vi "Config.vi"() -> ()   [LabVIEW 2020]
uses:
  Global_Variable/Global.vi
  <vilib>/Utility/config.llb/NI_LVConfig.lvlib
  Libraries/S7/S7.lvlib
panel:
  in  "扭矩偏移":string[][](table)=[["mm"], ["mm/s"], ["mm"], ["mm/s"]]
  in  "选项卡控件":enum32{"输入轴", "静态标定", "可信度检测", "传感器特性"}(tab)
  in  "左工位输入轴参数":string[][](table)=[["mm"], ["mm/s"], ["mm"], ["mm/s"]]
  in  "右工位输入轴参数":string[][](table)=[["mm"], ["mm/s"], ["mm"], ["mm/s"]]
  in  "静态标定判定":string[][](table)=[["mm"], ["mm/s"], ["mm"], ["mm/s"]]
  in  "跳过优化":bool
  in  "8点复测":bool
  in  "动态优化复测":bool
  in  "可信度检测参数":string[][](table)=[["mm/s"], ["°"], ["mm/s"]]
  in  "动态优化判定":string[][](table)=[["%"], ["%"], ["%"], ["%"]]
  in  "复检参数":string[][](table)=[["°/s"], ["Nm"], ["°"], ["°"], ["°"], ["°"]]
  in  "判定参数":string[][](table)=[["%", "", ""], ["%", "", ""], ["%", "", ""], ["%", "", ""], ["%", "", ""], ["%", "", ""], ["%", "", ""], ["%", "", ""], ["%", "", ""], ["Nm", "", ""], ["%", "", ""], ["%", "", ""], ["%", "", ""], ["%", "", ""]]
  in  "可信度检测":bool
  in  "传感器特性":bool
  in  "程序固化":bool
  in  "静态标定":bool
  in  "产品型号":string(combo)
  in  "删除":bool
  in  "确定":bool
  in  "添加":bool
  in  "退出":bool
  in  "更新":bool
  # "传感器对中台"
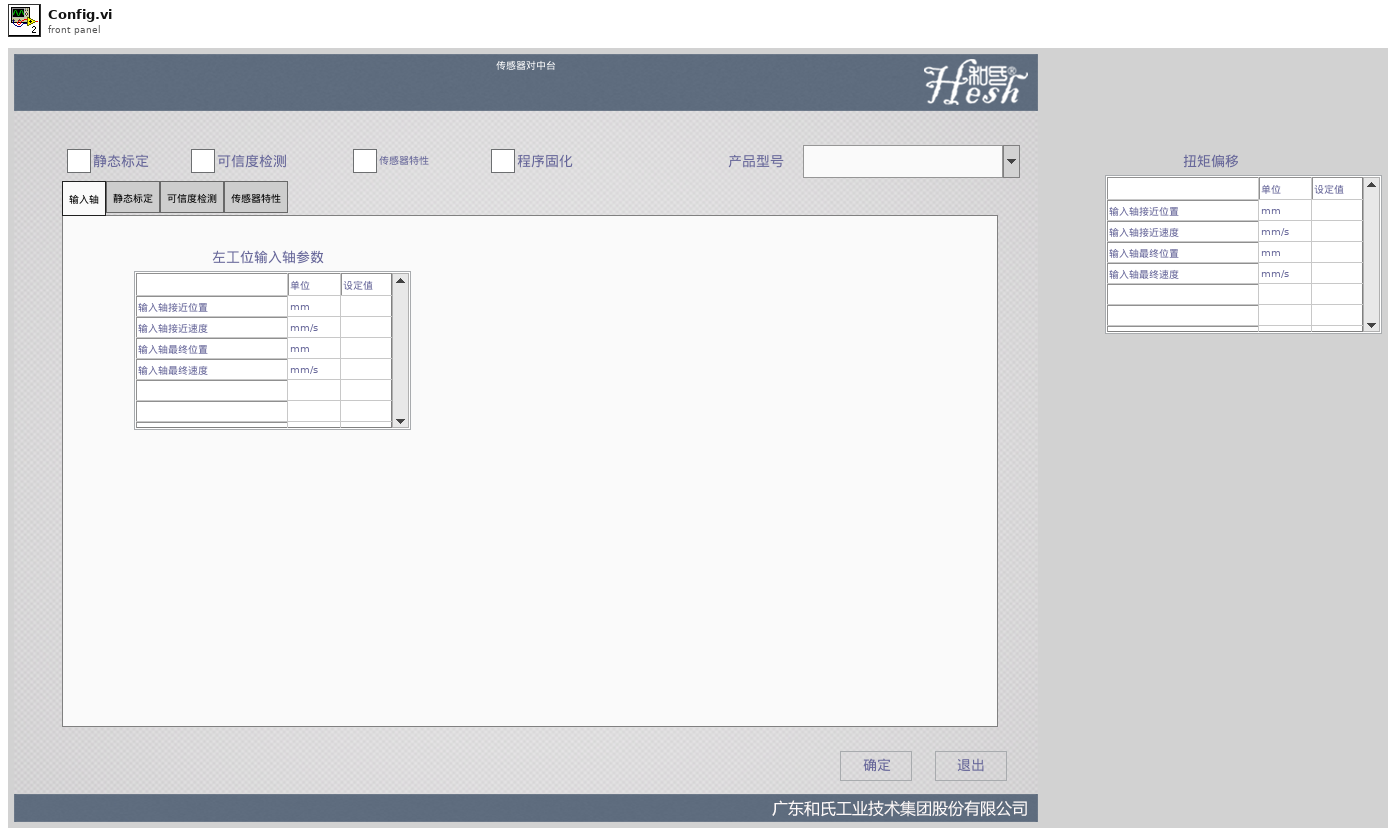
[diagram p1: front panel]
types:
  T1 = enum8{"Enabled", "Disabled", "Disabled and Grayed Out"}
  T2 = typedef "检测CTR.xctl/检测CTR数据.ctl" = enum16{"Idle", "Runing", "Pass", "Faild", "Skip"}
  T3 = cluster{"操作员编号":string, "操作员姓名":string, "操作员权限":string, "联机模式":enum16{"单机", "追溯"}}
  T4 = typedef "NI_LVConfig.lvlib/Config Data RefNum.ctl" = refnum<k1>
  T5 = cluster{"[0]":cluster{string, dbl, dbl}, "[1]":cluster{string, dbl, dbl}, "[2]":cluster{string, dbl, dbl}, "[3]":cluster{string, dbl, dbl}, "[4]":cluster{string, dbl, dbl}}
  T6 = cluster{"[0]":dbl, "[1]":dbl, "[2]":dbl, "[3]":dbl, "[4]":dbl, "[5]":dbl, "[6]":dbl}
  T7 = cluster{"[0]":cluster{string, dbl, dbl}, "[1]":cluster{string, dbl, dbl}, "[2]":cluster{string, dbl, dbl}, "[3]":cluster{string, dbl, dbl}, "[4]":cluster{string, dbl, dbl}, "[5]":cluster{string, dbl, dbl}, "[6]":cluster{string, dbl, dbl}, "[7]":cluster{string, dbl, dbl}, "[8]":cluster{string, dbl, dbl}, "[9]":cluster{string, dbl, dbl}, "[10]":cluster{string, dbl, dbl}, "[11]":cluster{string, dbl, dbl}, "[12]":cluster{string, dbl, dbl}, "[13]":cluster{string, dbl, dbl}, "[14]":cluster{string, dbl, dbl}, "[15]":cluster{string, dbl, dbl}, "[16]":cluster{string, dbl, dbl}, "[17]":cluster{string, dbl, dbl}, "[18]":cluster{string, dbl, dbl}, "[19]":cluster{string, dbl, dbl}}
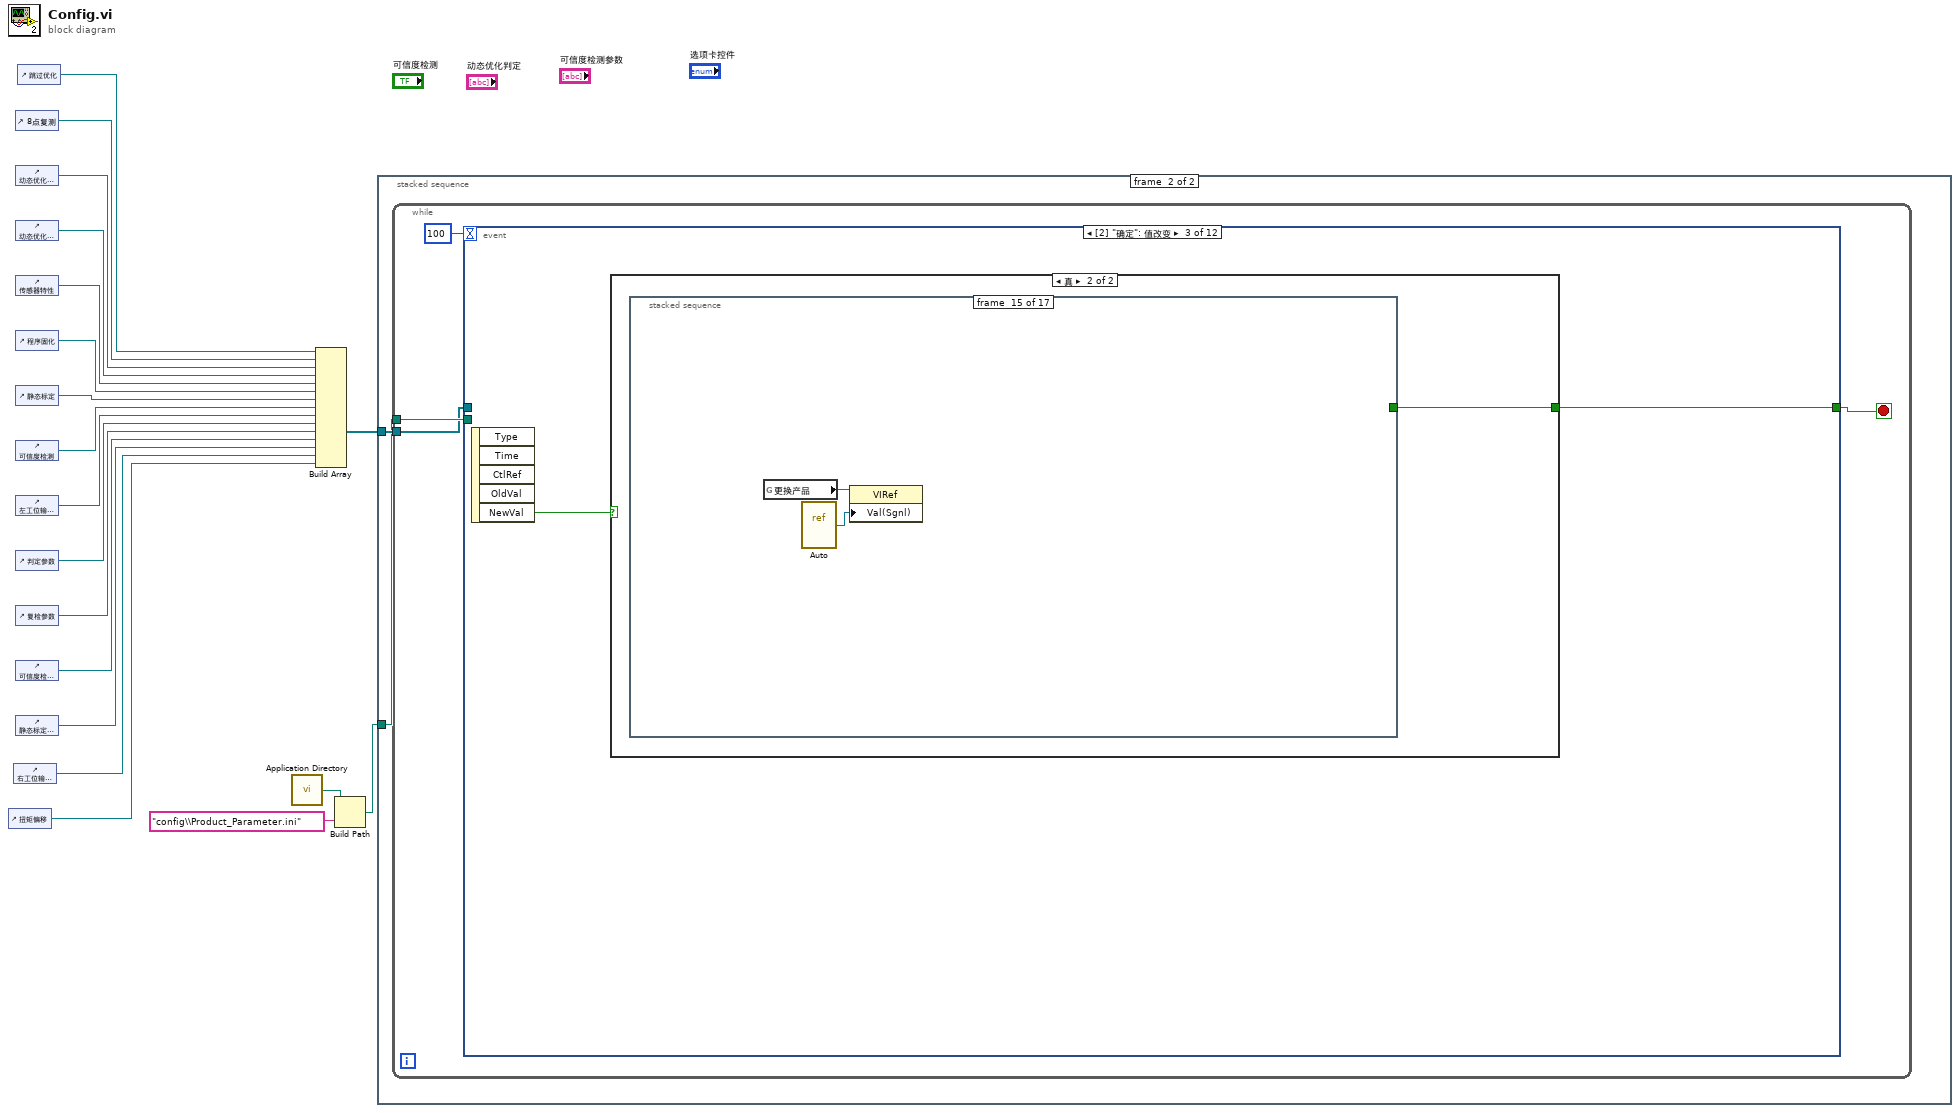
[diagram p0: block diagram]
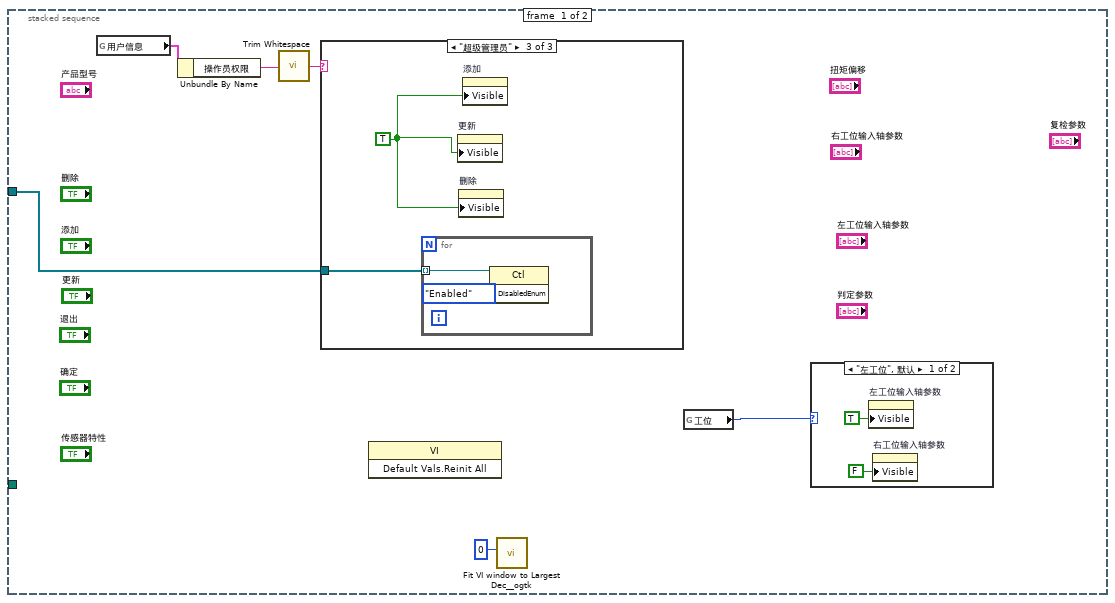
[diagram p2: hidden frame]
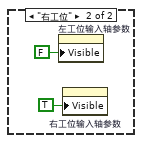
[diagram p3: hidden frame]
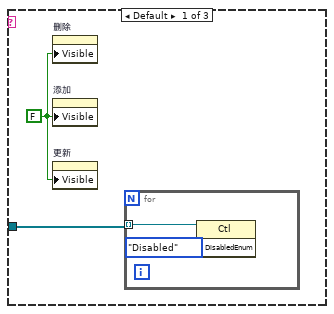
[diagram p4: hidden frame]
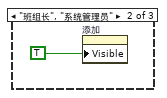
[diagram p5: hidden frame]
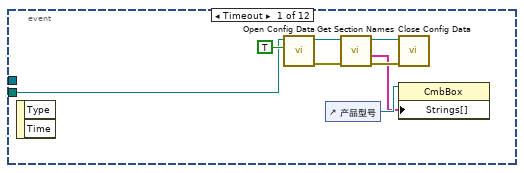
[diagram p6: hidden frame]
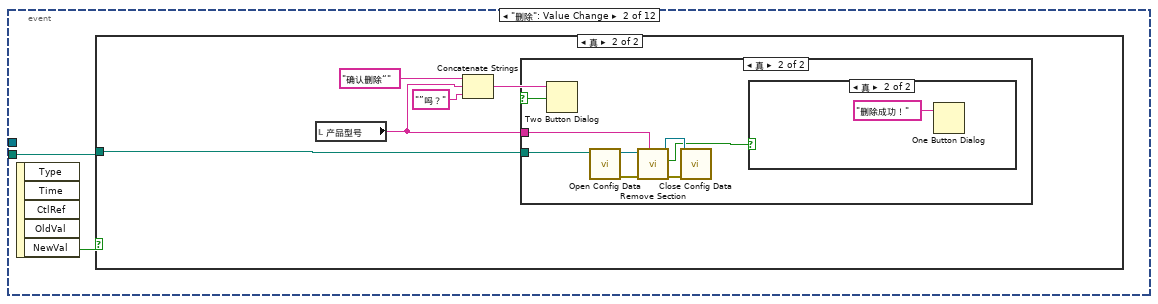
[diagram p7: hidden frame]
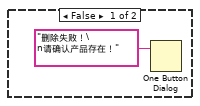
[diagram p10: hidden frame]
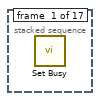
[diagram p12: hidden frame]
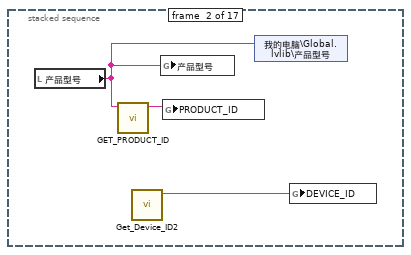
[diagram p13: hidden frame]
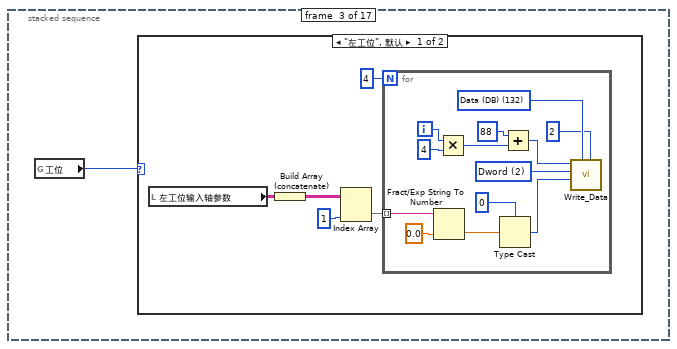
[diagram p14: hidden frame]
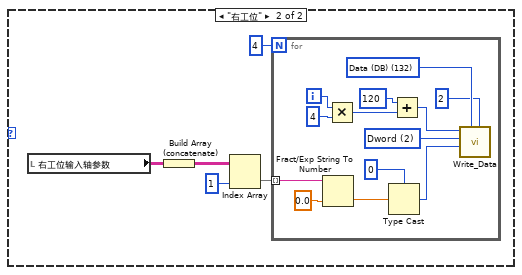
[diagram p15: hidden frame]
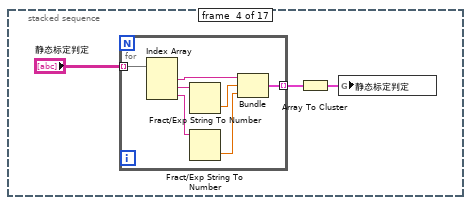
[diagram p16: hidden frame]
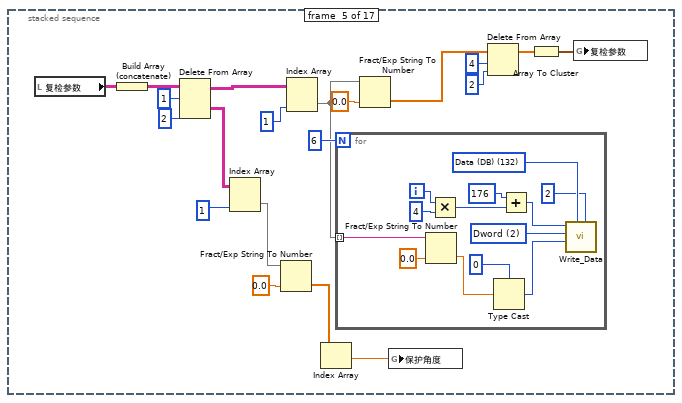
[diagram p17: hidden frame]
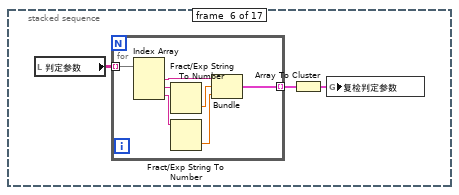
[diagram p18: hidden frame]
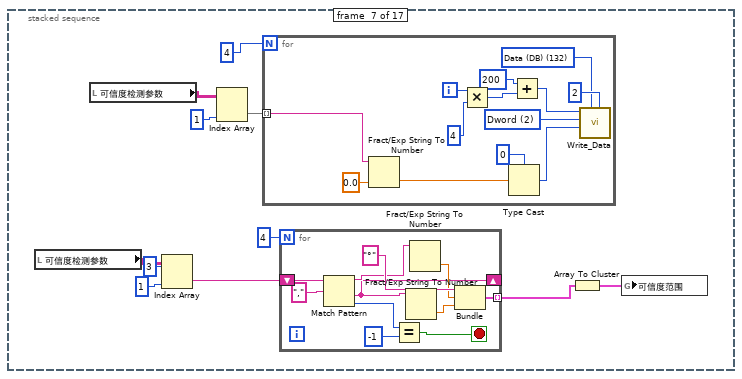
[diagram p19: hidden frame]
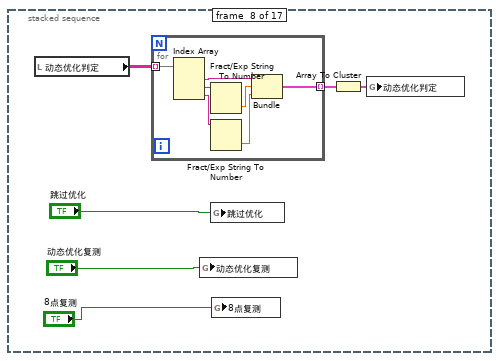
[diagram p20: hidden frame]
diagram:
  n1 = control-ref of="扭矩偏移"() -> (w1:refnum<vi>)
  n2 = control-ref of="右工位输入轴参数"() -> (w2:refnum<vi>)
  n3 = control-ref of="8点复测"() -> (w4:refnum<vi>)
  n4 = control-ref of="动态优化复测"() -> (w5:refnum<vi>)
  n5 = control-ref of="动态优化判定"() -> (w6:refnum<vi>)
  n6 = control-ref of="传感器特性"() -> (w11:refnum<vi>)
  n7 = control-ref of="程序固化"() -> (w12:refnum<vi>)
  n8 = control-ref of="静态标定"() -> (w13:refnum<vi>)
  n9 = control-ref of="可信度检测"() -> (w9:refnum<vi>)
  n10 = control-ref of="左工位输入轴参数"() -> (w14:refnum<vi>)
  n11 = control-ref of="判定参数"() -> (w15:refnum<vi>)
  n12 = control-ref of="复检参数"() -> (w10:refnum<vi>)
  n13 = control-ref of="可信度检测参数"() -> (w8:refnum<vi>)
  n14 = control-ref of="静态标定判定"() -> (w7:refnum<vi>)
  n15 = control-ref of="跳过优化"() -> (w3:refnum<vi>)
  n16 = call <vilib>:"Application Directory.vi"() -> ("Application Directory"=w18:path)
  n17 = Build Array(w3, w4, w5, w6, w11, w12, w13, w9, w14, w15, w10, w8, w7, w2, w1) -> (w19:refnum<vi>[])
  n18 = Build Path(base path=w18, name or relative path="config\\Product_Parameter.ini" ("名称或相对路径")) -> (appended path=w16:path)
  n19 = stacked-sequence {
    tunnel: w19 -> [w20 w40]
    tunnel: w16 -> [_ w39]
    frame #0 {
      n20 = global read "用户信息.vi" "用户信息"() -> (w23:T3)
      n21 = Unbundle By Name(w23) -> ("操作员权限"=w22:string)
      n22 = call <vilib>:"Trim Whitespace.vi"("string"=w22) -> ("trimmed string"=w25:string)  [unwired: 1 in]
      n23 = case shown="\"超级管理员\"" w25 {
        tunnel: w20 -> [w30 _ w35]
        frame Default {
          w31 = FALSE ("可见")
          n24 = property on="删除" class="Bool (严格)"("Visible"=w31) -> ()  [unwired: 2 in, 2 out]
          n25 = property on="添加" class="Bool (严格)"("Visible"=w31) -> ()  [unwired: 2 in, 2 out]
          n26 = property on="更新" class="Bool (严格)"("Visible"=w31) -> ()  [unwired: 2 in, 2 out]
          n27 = for {
            tunnel: w30 -> [w33] mode=indexing
            n28 = property class="Ctl"(reference=w33, "DisabledEnum"=T1."Disabled" ("禁用")) -> ()  [unwired: 1 in, 2 out]
          }
        }
        frame "班组长", "系统管理员" {
          n29 = property on="添加" class="Bool (严格)"("Visible"=TRUE ("可见")) -> ()  [unwired: 2 in, 2 out]
        }
        frame "超级管理员" {
          w36 = TRUE
          n30 = for {
            tunnel: w35 -> [w38] mode=indexing
            n31 = property class="Ctl"(reference=w38, "DisabledEnum"=T1."Enabled" ("禁用")) -> ()  [unwired: 1 in, 2 out]
          }
          n32 = property on="更新" class="Bool (严格)"("Visible"=w36) -> ()  [unwired: 2 in, 2 out]
          n33 = property on="删除" class="Bool (严格)"("Visible"=w36) -> ()  [unwired: 2 in, 2 out]
          n34 = property on="添加" class="Bool (严格)"("Visible"=w36) -> ()  [unwired: 2 in, 2 out]
        }
      }
      n35 = invoke class="VI" method="Default Vals.Reinit All"() -> ()  [unwired: 3 in, 3 out]
      n36 = call <userlib>:"Fit VI window to Largest Dec__ogtk.vi"("border spacing (2 px)"=0) -> ()  [unwired: 5 in, 2 out]
      n37 = global read "Global.vi" "工位"() -> (w21:enum16{"左工位", "右工位"})
      n38 = case shown="\"左工位\", 默认" w21 {
        frame "左工位", Default {
          n39 = property on="左工位输入轴参数" class="Tbl (严格)"("Visible"=TRUE ("可见")) -> ()  [unwired: 2 in, 2 out]
          n40 = property on="右工位输入轴参数" class="Tbl (严格)"("Visible"=FALSE ("可见")) -> ()  [unwired: 2 in, 2 out]
        }
        frame "右工位" {
          n41 = property on="左工位输入轴参数" class="Tbl (严格)"("Visible"=FALSE ("可见")) -> ()  [unwired: 2 in, 2 out]
          n42 = property on="右工位输入轴参数" class="Tbl (严格)"("Visible"=TRUE ("可见")) -> ()  [unwired: 2 in, 2 out]
        }
      }
    }
    frame #1 {
      n43 = while {
        tunnel: w39 -> [w44]
        tunnel: w40 -> [w42]
        stop <- w43 stop-if-true
        n44 = event shown="[2] \"确定\": 值改变" {
          selector: _ -> [_ _ _ _ _ _ _ _ _ _ _ _]
          dyn-events: _ -> [_ _ _ _ _ _ _ _ _ _ _ _]
          timeout: 100 -> [_ _ _ _ _ _ _ _ _ _ _ _]
          tunnel: w44 -> [w47 w54 _ _ _ _ _ w271 w299 _ w315 _]
          tunnel: [_ _ w70 _ _ _ _ _ _ TRUE _ TRUE] -> w43
          tunnel: w42 -> [_ _ _ _ _ _ _ w272 w300 _ w314 _]
          event Timeout {
            n45 = event-data() -> ()  [unwired: 1 in, 2 out]
            n46 = call <vilib>:"Open Config Data.vi"("create file if necessary (T)"=TRUE, "configuration file path"=w47) -> ("error out"=w49:errorcluster, "refnum"=w48:T4)  [unwired: 7 in, 1 out]
            n47 = control-ref of="产品型号"() -> (w46:refnum<vi>)
            n48 = call <vilib>:"Get Section Names.vi"("error in (no error)"=w49, "refnum"=w48) -> ("error out"=w51:errorcluster, "section names"=w45:string[], "refnum out"=w50:T4)  [unwired: 7 in]
            n49 = call <vilib>:"Close Config Data.vi"("error in (no error)"=w51, "refnum"=w50) -> ()  [unwired: 8 in, 2 out]
            n50 = property on="属性节点" class="CmbBox"(reference=w46, "Strings[]"=w45) -> ()  [unwired: 1 in, 2 out]
          }
          event "删除": Value Change {
            n51 = event-data() -> ("NewVal"=w53:bool)  [unwired: 1 in, 4 out]
            n52 = case shown="真" w53 {
              tunnel: w54 -> [_ w56]
              frame False {
              }
              frame True {
                n53 = local read "产品型号"() -> (w55:string)
                n54 = Concatenate Strings("确认删除“", w55, "”吗？") -> (w58:string)
                n55 = Two Button Dialog(message=w58) -> (T button?=w57:bool)  [unwired: 2 in]
                n56 = case shown="真" w57 {
                  tunnel: w56 -> [_ w62]
                  tunnel: w55 -> [_ w61]
                  frame False {
                  }
                  frame True {
                    n57 = call <vilib>:"Open Config Data.vi"("configuration file path"=w62) -> ("error out"=w64:errorcluster, "refnum"=w67:T4)  [unwired: 8 in, 1 out]
                    n58 = call <vilib>:"Remove Section.vi"("section"=w61, "error in (no error)"=w64, "refnum"=w67) -> ("error out"=w66:errorcluster, "section exists?"=w63:bool, "refnum out"=w65:T4)  [unwired: 6 in]
                    n59 = call <vilib>:"Close Config Data.vi"("error in (no error)"=w66, "refnum"=w65) -> ()  [unwired: 8 in, 2 out]
                    n60 = case shown="真" w63 {
                      frame False {
                        n61 = One Button Dialog(message="删除失败！\n请确认产品存在！" ("消息")) -> ()  [unwired: 1 in, 1 out]
                      }
                      frame True {
                        n62 = One Button Dialog(message="删除成功！" ("消息")) -> ()  [unwired: 1 in, 1 out]
                      }
                    }
                  }
                }
              }
            }
          }
          event "确定": Value Change {
            n63 = event-data() -> ("NewVal"=w71:bool)  [unwired: 1 in, 4 out]
            n64 = case shown="真" w71 {
              tunnel: [_ w72] -> w70
              frame False {
              }
              frame True {
                n65 = stacked-sequence {
                  tunnel: [_ _ _ _ _ _ _ _ _ _ _ _ _ _ _ _ TRUE] -> w72
                  frame #0 {
                    n66 = call <vilib>:"Set Busy.vi"() -> ()  [unwired: 10 in, 2 out]
                  }
                  frame #1 {
                    n67 = local read "产品型号"() -> (w74:string)
                    n68 = call "GET_PRODUCT_ID.vi"("PRODFUCT_NAME"=w74) -> ("PRODUCT_ID"=w75:string)  [unwired: 10 in]
                    n69 = call "Get_Device_ID2.vi"() -> ("Device_ID"=w73:string)  [unwired: 10 in, 1 out]
                    n70 = global write "Global.vi" "产品型号"(w74) -> ()
                    n71 = global write "追溯Global.vi" "PRODUCT_ID"(w75) -> ()
                    n72 = shared-variable "我的电脑\\Global.lvlib\\产品型号"(w74) -> ()  [unwired: 1 in, 1 out]
                    n73 = global write "追溯Global.vi" "DEVICE_ID"(w73) -> ()
                  }
                  frame #2 {
                    n74 = global read "Global.vi" "工位"() -> (w76:enum16{"左工位", "右工位"})
                    n75 = case shown="\"左工位\", 默认" w76 {
                      frame "左工位", Default {
                        n76 = local read "左工位输入轴参数"() -> (w79:string[][])
                        n77 = Build Array (concatenate)(w79) -> (w78:string[][])
                        n78 = Index Array(array=w78, index (col)=1 ("禁用的索引 (列)")) -> (element=w81:string[])  [unwired: 1 in]
                        n79 = for {
                          N: 4 -> [_]
                          tunnel: w81 -> [w90] mode=indexing
                          i -> [w84]
                          w92 = u16 2 items=["byte", "word", "Dword"] ("数据类型")
                          w94 = u8 132 items=["I/O (P)"=128, "Input (I)"=129, "Output (Q)"=130, "Bit Memory (M)"=131, "Data (DB)"=132, "Instance Data (DI)"=133, "Local Data (L)"=134, "Predecessor Local Data (VL)"=135] ("寄存器类型")
                          n80 = Fract/Exp String To Number(string=w90, default (0 dbl)=sgl 0.0) -> (number=w88:sgl)  [unwired: 2 in, 1 out]
                          n81 = Multiply(x=w84, y=4) -> (x*y=w85:i32)
                          n82 = Type Cast(type=u32 0 ("写入地址"), x=w88) -> (*(type *) &x=w87:u32)
                          n83 = Add(x=u32 88 ("写入地址"), y=w85) -> (x+y=w82:u32)
                          n84 = call "Write_Data.vi"("DB #"=u16 2, "寄存器类型"=w94, "写入数据"=w87, "数据类型"=w92, "写入地址"=w82) -> ()  [unwired: 4 in, 3 out]
                        }
                      }
                      frame "右工位" {
                        n85 = local read "右工位输入轴参数"() -> (w98:string[][])
                        n86 = Build Array (concatenate)(w98) -> (w97:string[][])
                        n87 = Index Array(array=w97, index (col)=1 ("禁用的索引 (列)")) -> (element=w99:string[])  [unwired: 1 in]
                        n88 = for {
                          N: 4 -> [_]
                          tunnel: w99 -> [w108] mode=indexing
                          i -> [w102]
                          w110 = u16 2 items=["byte", "word", "Dword"] ("数据类型")
                          w112 = u8 132 items=["I/O (P)"=128, "Input (I)"=129, "Output (Q)"=130, "Bit Memory (M)"=131, "Data (DB)"=132, "Instance Data (DI)"=133, "Local Data (L)"=134, "Predecessor Local Data (VL)"=135] ("寄存器类型")
                          n89 = Fract/Exp String To Number(string=w108, default (0 dbl)=sgl 0.0) -> (number=w106:sgl)  [unwired: 2 in, 1 out]
                          n90 = Multiply(x=w102, y=4) -> (x*y=w103:i32)
                          n91 = Type Cast(type=u32 0 ("写入地址"), x=w106) -> (*(type *) &x=w105:u32)
                          n92 = Add(x=u32 120 ("写入地址"), y=w103) -> (x+y=w100:u32)
                          n93 = call "Write_Data.vi"("DB #"=u16 2, "寄存器类型"=w112, "写入数据"=w105, "数据类型"=w110, "写入地址"=w100) -> ()  [unwired: 4 in, 3 out]
                        }
                      }
                    }
                  }
                  frame #3 {
                    n94 = for {
                      tunnel: "静态标定判定" -> [w122] mode=indexing
                      tunnel: [w116] -> w114 mode=indexing
                      n95 = Index Array(array=w122) -> (element #1=w119:string, element #2=w121:string, element #3=w120:string)  [unwired: 3 in]
                      n96 = Fract/Exp String To Number(string=w121) -> (number=w118:dbl)  [unwired: 3 in, 1 out]
                      n97 = Fract/Exp String To Number(string=w120) -> (number=w117:dbl)  [unwired: 3 in, 1 out]
                      n98 = Bundle(w119, w118, w117) -> (w116:cluster{string, dbl, dbl})  [unwired: 1 in]
                    }
                    n99 = Array To Cluster(array=w114) -> (cluster=w113:T5)
                    n100 = global write "Global.vi" "静态标定判定"(w113) -> ()
                  }
                  frame #4 {
                    n101 = local read "复检参数"() -> (w142:string[][])
                    n102 = Build Array (concatenate)(w142) -> (w132:string[][])
                    n103 = Delete From Array(array=w132, length=1 ("长度"), index (row)=2 ("索引 (行)")) -> (deleted portion=w128:string[][], array with subset deleted=w129:string[][])  [unwired: 1 in]
                    n104 = Index Array(array=w128, index (col)=1 ("禁用的索引 (列)")) -> (element=w125:string[])  [unwired: 1 in]
                    n105 = Fract/Exp String To Number(string=w125, default (0 dbl)=0.0) -> (number=w124:dbl[])  [unwired: 2 in, 1 out]
                    n106 = Index Array(array=w129, index (col)=1 ("禁用的索引 (列)")) -> (element=w138:string[])  [unwired: 1 in]
                    n107 = Index Array(array=w124) -> (element=w123:dbl)  [unwired: 1 in]
                    n108 = for {
                      N: 6 -> [_]
                      tunnel: w138 -> [w151] mode=indexing
                      i -> [w145]
                      w153 = u16 2 items=["byte", "word", "Dword"] ("数据类型")
                      w155 = u8 132 items=["I/O (P)"=128, "Input (I)"=129, "Output (Q)"=130, "Bit Memory (M)"=131, "Data (DB)"=132, "Instance Data (DI)"=133, "Local Data (L)"=134, "Predecessor Local Data (VL)"=135] ("寄存器类型")
                      n109 = Fract/Exp String To Number(string=w151, default (0 dbl)=sgl 0.0) -> (number=w149:sgl)  [unwired: 2 in, 1 out]
                      n110 = Multiply(x=w145, y=4) -> (x*y=w146:i32)
                      n111 = Type Cast(type=u32 0 ("写入地址"), x=w149) -> (*(type *) &x=w148:u32)
                      n112 = Add(x=u32 176 ("写入地址"), y=w146) -> (x+y=w143:u32)
                      n113 = call "Write_Data.vi"("DB #"=u16 2, "寄存器类型"=w155, "写入数据"=w148, "数据类型"=w153, "写入地址"=w143) -> ()  [unwired: 4 in, 3 out]
                    }
                    n114 = Fract/Exp String To Number(string=w138, default (0 dbl)=0.0) -> (number=w137:dbl[])  [unwired: 2 in, 1 out]
                    n115 = global write "Global.vi" "保护角度"(w123) -> ()
                    n116 = Delete From Array(array=w137, length=4 ("长度"), index=2 ("索引")) -> (array with subset deleted=w135:dbl[])  [unwired: 1 out]
                    n117 = Array To Cluster(array=w135) -> (cluster=w136:T6)
                    n118 = global write "Global.vi" "复检参数"(w136) -> ()
                  }
                  frame #5 {
                    n119 = local read "判定参数"() -> (w158:string[][])
                    n120 = for {
                      tunnel: w158 -> [w165] mode=indexing
                      tunnel: [w159] -> w157 mode=indexing
                      n121 = Index Array(array=w165) -> (element #1=w162:string, element #2=w164:string, element #3=w163:string)  [unwired: 3 in]
                      n122 = Fract/Exp String To Number(string=w164) -> (number=w161:dbl)  [unwired: 3 in, 1 out]
                      n123 = Fract/Exp String To Number(string=w163) -> (number=w160:dbl)  [unwired: 3 in, 1 out]
                      n124 = Bundle(w162, w161, w160) -> (w159:cluster{string, dbl, dbl})  [unwired: 1 in]
                    }
                    n125 = Array To Cluster(array=w157) -> (cluster=w156:T7)
                    n126 = global write "Global.vi" "复检判定参数"(w156) -> ()
                  }
                  frame #6 {
                    n127 = local read "可信度检测参数"() -> (w171:string[][])
                    n128 = local read "可信度检测参数"() -> (w176:string[][])
                    n129 = Index Array(array=w171, index (row)=3 ("禁用的索引 (行)"), index (col)=1 ("索引")) -> (element=w170:string)
                    n130 = Index Array(array=w176, index (col)=1 ("索引")) -> (element=w175:string[])  [unwired: 1 in]
                    n131 = for {
                      N: 4 -> [_]
                      tunnel: w175 -> [w188] mode=indexing
                      i -> [w190]
                      w192 = u16 2 items=["byte", "word", "Dword"] ("数据类型")
                      w193 = u8 132 items=["I/O (P)"=128, "Input (I)"=129, "Output (Q)"=130, "Bit Memory (M)"=131, "Data (DB)"=132, "Instance Data (DI)"=133, "Local Data (L)"=134, "Predecessor Local Data (VL)"=135] ("寄存器类型")
                      n132 = Fract/Exp String To Number(string=w188, default (0 dbl)=sgl 0.0 ("默认(0 DBL)")) -> (number=w191:sgl)  [unwired: 2 in, 1 out]
                      n133 = Multiply(x=w190, y=4) -> (x*y=w199:i32)
                      n134 = Type Cast(type=u32 0 ("写入地址"), x=w191) -> (*(type *) &x=w198:u32)
                      n135 = Add(x=u32 200 ("写入地址"), y=w199) -> (x+y=w200:u32)
                      n136 = call "Write_Data.vi"("DB #"=u16 2, "寄存器类型"=w193, "写入数据"=w198, "数据类型"=w192, "写入地址"=w200) -> ()  [unwired: 4 in, 3 out]
                    }
                    n137 = for {
                      N: 4 -> [_]
                      shift-right: [w179] -> _
                      shift-left: w170 -> [w187]
                      tunnel: [w177] -> w167 mode=indexing
                      stop <- w183 stop-if-true
                      n138 = Match Pattern(string=w187, regular expression="," ("正则表达式")) -> (before substring=w181:string, after substring=w179:string, offset past match=w185:i32)  [unwired: 1 in, 1 out]
                      n139 = Equal?(x=w185, y=-1) -> (x = y?=w183:bool)
                      n140 = Fract/Exp String To Number(string=w179) -> (number=w178:dbl)  [unwired: 3 in, 1 out]
                      n141 = Fract/Exp String To Number(string=w181) -> (number=w180:dbl)  [unwired: 3 in, 1 out]
                      n142 = Bundle("正则表达式"="°", w180, w178) -> (w177:cluster{"正则表达式":string, dbl, dbl})  [unwired: 1 in]
                    }
                    n143 = Array To Cluster(array=w167) -> (cluster=w166:cluster{"[0]":cluster{"正则表达式":string, dbl, dbl}})
                    n144 = global write "Global.vi" "可信度范围"(w166) -> ()
                  }
                  frame #7 {
                    n145 = local read "动态优化判定"() -> (w206:string[][])
                    n146 = for {
                      tunnel: w206 -> [w213] mode=indexing
                      tunnel: [w207] -> w205 mode=indexing
                      n147 = Index Array(array=w213) -> (element #1=w210:string, element #2=w212:string, element #3=w211:string)  [unwired: 3 in]
                      n148 = Fract/Exp String To Number(string=w212) -> (number=w209:dbl)  [unwired: 3 in, 1 out]
                      n149 = Fract/Exp String To Number(string=w211) -> (number=w208:dbl)  [unwired: 3 in, 1 out]
                      n150 = Bundle(w210, w209, w208) -> (w207:cluster{string, dbl, dbl})  [unwired: 1 in]
                    }
                    n151 = global write "Global.vi" "动态优化复测"("动态优化复测") -> ()
                    n152 = global write "Global.vi" "跳过优化"("跳过优化") -> ()
                    n153 = global write "Global.vi" "8点复测"("8点复测") -> ()
                    n154 = Array To Cluster(array=w205) -> (cluster=w204:T5)
                    n155 = global write "Global.vi" "动态优化判定"(w204) -> ()
                  }
                  frame #8 {
                    n156 = local read "静态标定"() -> (w214:bool)
                    n157 = case shown="假" w214 {
                      frame False {
                        n158 = global read "Global.vi" "静态标定引用句柄"() -> (w216:refnum<vi>)
                        n159 = property class="检测CTR"(reference=w216, "Value"=检测CTR数据."Skip" ("Data")) -> ()  [unwired: 1 in, 2 out]
                      }
                      frame True {
                        n160 = global read "Global.vi" "静态标定引用句柄"() -> (w218:refnum<vi>)
                        n161 = property class="检测CTR"(reference=w218, "Value"=检测CTR数据."Idle" ("Data")) -> ()  [unwired: 1 in, 2 out]
                      }
                    }
                  }
                  frame #9 {
                    n162 = local read "程序固化"() -> (w219:bool)
                    n163 = case shown="假" w219 {
                      frame False {
                        n164 = global read "Global.vi" "程序固化引用句柄"() -> (w221:refnum<vi>)
                        n165 = property class="检测CTR"(reference=w221, "Value"=检测CTR数据."Skip" ("Data")) -> ()  [unwired: 1 in, 2 out]
                      }
                      frame True {
                        n166 = global read "Global.vi" "程序固化引用句柄"() -> (w223:refnum<vi>)
                        n167 = property class="检测CTR"(reference=w223, "Value"=检测CTR数据."Idle" ("Data")) -> ()  [unwired: 1 in, 2 out]
                      }
                    }
                  }
                  frame #10 {
                    n168 = local read "传感器特性"() -> (w224:bool)
                    n169 = case shown="假" w224 {
                      frame False {
                        n170 = global read "Global.vi" "传感器特性用句柄"() -> (w226:refnum<vi>)
                        n171 = property class="检测CTR"(reference=w226, "Value"=检测CTR数据."Skip" ("Data")) -> ()  [unwired: 1 in, 2 out]
                      }
                      frame True {
                        n172 = global read "Global.vi" "传感器特性用句柄"() -> (w227:refnum<vi>)
                        n173 = property class="检测CTR"(reference=w227, "Value"=检测CTR数据."Idle" ("Data")) -> ()  [unwired: 1 in, 2 out]
                      }
                    }
                  }
                  frame #11 {
                    n174 = local read "跳过优化"() -> (w229:bool)
                    n175 = local read "可信度检测"() -> (w230:bool)
                    n176 = case shown="假" w230 {
                      frame False {
                        n177 = global read "Global.vi" "可信度检测引用句柄"() -> (w235:refnum<vi>)
                        n178 = property class="检测CTR"(reference=w235, "Value"=检测CTR数据."Skip" ("Data")) -> ()  [unwired: 1 in, 2 out]
                      }
                      frame True {
                        n179 = global read "Global.vi" "可信度检测引用句柄"() -> (w237:refnum<vi>)
                        n180 = property class="检测CTR"(reference=w237, "Value"=检测CTR数据."Idle" ("Data")) -> ()  [unwired: 1 in, 2 out]
                      }
                    }
                    n181 = case shown="真" w229 {
                      frame False {
                        n182 = global read "Global.vi" "动态优化引用句柄"() -> (w232:refnum<vi>)
                        n183 = property class="检测CTR"(reference=w232, "Value"=检测CTR数据."Idle" ("Data")) -> ()  [unwired: 1 in, 2 out]
                      }
                      frame True {
                        n184 = global read "Global.vi" "动态优化引用句柄"() -> (w233:refnum<vi>)
                        n185 = property class="检测CTR"(reference=w233, "Value"=检测CTR数据."Skip" ("Data")) -> ()  [unwired: 1 in, 2 out]
                      }
                    }
                  }
                  frame #12 {
                    n186 = local read "可信度检测"() -> (w240:bool)
                    n187 = local read "传感器特性"() -> (w242:bool)
                    n188 = local read "静态标定"() -> (w241:bool)
                    n189 = local read "程序固化"() -> (w239:bool)
                    n190 = Build Array(w241, w240, w242, w239) -> (w243:bool[])
                    n191 = global write "Global.vi" "试验项目"(w243) -> ()
                  }
                  frame #13 {
                    n192 = call <vilib>:"Unset Busy.vi"() -> ()  [unwired: 11 in, 1 out]
                  }
                  frame #14 {
                    n193 = global read "Global.vi" "更换产品"() -> (w245:refnum<vi>)
                    n194 = vi-ref "Auto.vi"() -> (w244:refnum<vi>)
                    n195 = property class="VIRef"(reference=w245, "Val(Sgnl)"=w244) -> ()  [unwired: 1 in, 2 out]
                  }
                  frame #15 {
                    w246 = "参数装载成功！" ("消息")
                    n196 = call "浮动通知.vi"("通知内容"=w246) -> ()  [unwired: 11 in]
                    n197 = One Button Dialog(message=w246) -> ()  [unwired: 1 in, 1 out]
                  }
                  frame #16 {
                    n198 = control-ref of="本VI"() -> (w247:refnum<vi>)
                    n199 = invoke class="VI" method="FP.Close"(reference=w247) -> ()  [unwired: 2 in, 3 out]
                  }
                }
              }
            }
          }
          event "静态标定": Value Change {
            n200 = event-data() -> ("NewVal"=w249:bool)  [unwired: 1 in]
            n201 = case shown="假" w249 {
              selector: w249 -> [w250 _]
              frame False {
                n202 = local write "程序固化"(w250) -> ()
              }
              frame True {
              }
            }
          }
          event "程序固化": Value Change {
            n203 = event-data() -> ("NewVal"=w251:bool)  [unwired: 1 in]
            n204 = case shown="真" w251 {
              selector: w251 -> [_ w252]
              frame False {
              }
              frame True {
                n205 = local write "静态标定"(w252) -> ()
              }
            }
          }
          event "可信度检测": Value Change {
            n206 = event-data() -> ("NewVal"=w253:bool)  [unwired: 1 in, 5 out]
            n207 = case shown="真" w253 {
              selector: w253 -> [_ w254]
              frame False {
              }
              frame True {
                n208 = local write "可信度检测"(w254) -> ()
              }
            }
          }
          event "复检参数": Value Change {
            (unwired) "1"
            n209 = event-data() -> ()  [unwired: 1 in, 6 out]
            n210 = local read "复检参数"() -> (w269:string[][])
            n211 = Index Array(array=w269) -> (element=w268:string[])  [unwired: 2 in]
            n212 = Index Array(array=w268, index=1 ("索引")) -> (element=w267:string)
            n213 = Fract/Exp String To Number(string=w267) -> (number=w259:dbl)  [unwired: 3 in, 1 out]
            n214 = Greater Or Equal?(x=w259, y=sgl 1.0) -> (x >= y?=w266:bool)
            n215 = Number To Fractional String(number=w259, precision (6)=i16 1 ("精度(6)")) -> (F-format string=w256:string)  [unwired: 2 in]
            n216 = Select(t="1", s=w266, f=w256) -> (s? t:f=w260:string)
            n217 = local read "复检参数"() -> (w264:string[][])
            n218 = Build Array(w260) -> (w262:string[])
            n219 = Replace Array Subset(array=w264, new element=w262, index (col)=1 ("禁用的索引 (列)")) -> (w261:string[][])  [unwired: 1 in]
            n220 = local write "复检参数"(w261) -> ()
          }
          event "添加": Value Change {
            n221 = event-data() -> ("NewVal"=w270:bool)  [unwired: 1 in, 4 out]
            n222 = case shown="真" w270 {
              tunnel: w272 -> [_ w276]
              tunnel: w271 -> [_ w275]
              frame False {
              }
              frame True {
                n223 = call "产品添加提示：用户输入"() -> ("产品型号"=w273:string, "确定"=w274:bool)  [unwired: 17 in, 1 out]
                n224 = case shown="真" w274 {
                  tunnel: w276 -> [_ w279]
                  tunnel: w275 -> [_ w278]
                  tunnel: w273 -> [_ w277]
                  frame False {
                  }
                  frame True {
                    n225 = case shown="默认" w277 {
                      selector: w277 -> [_ w282]
                      tunnel: w279 -> [_ w285]
                      tunnel: w278 -> [_ w284]
                      frame "" {
                        n226 = One Button Dialog(message="产品名称不得为空!" ("text")) -> ()  [unwired: 1 in, 1 out]
                      }
                      frame Default {
                        n227 = property on="产品型号" class="CmbBox"() -> ("Strings[]"=w283:string[])  [unwired: 2 in, 2 out]
                        n228 = Search 1D Array(1D array=w283, element=w282) -> (index of element=w281:i32)  [unwired: 1 in]
                        n229 = case shown="-1" w281 {
                          tunnel: w285 -> [_ w289]
                          tunnel: w284 -> [_ w288]
                          tunnel: w282 -> [_ w287]
                          frame Default {
                            n230 = One Button Dialog(message="产品已存在！" ("消息")) -> ()  [unwired: 1 in, 1 out]
                          }
                          frame -1 {
                            n231 = stacked-sequence {
                              tunnel: w289 -> [w292 _]
                              tunnel: w288 -> [w291 _]
                              tunnel: w287 -> [w290 _]
                              frame #0 {
                                n232 = for {
                                tunnel: w292 -> [w295] mode=indexing
                                tunnel: w291 -> [w294]
                                tunnel: w290 -> [w293]
                                n233 = call "Read_Write ParaINI File.vi"("Mode"=enum16{"Read", "Write"}."Write", "Section"=w293, "Filepath"=w294, "Ctl Refnum"=w295) -> ()  [unwired: 7 in, 1 out]
                                }
                              }
                              frame #1 {
                                n234 = One Button Dialog(message="添加成功！" ("消息")) -> ()  [unwired: 1 in, 1 out]
                              }
                            }
                          }
                        }
                      }
                    }
                  }
                }
              }
            }
          }
          event "产品型号": Value Change {
            n235 = event-data() -> ("NewVal"=w298:string)  [unwired: 1 in, 4 out]
            n236 = stacked-sequence {
              tunnel: w300 -> [_ _ w304]
              tunnel: w299 -> [_ _ w303]
              tunnel: w298 -> [_ w302 _]
              frame #0 {
                n237 = control-ref of="本VI"() -> (w301:refnum<vi>)
                n238 = invoke class="VI" method="Default Vals.Reinit All"(reference=w301) -> ()  [unwired: 2 in, 3 out]
              }
              frame #1 {
                n239 = local write "产品型号"(w302) -> ()
              }
              frame #2 {
                n240 = for {
                  tunnel: w304 -> [w307] mode=indexing
                  tunnel: w303 -> [w306]
                  n241 = local read "产品型号"() -> (w305:string)
                  n242 = call "Read_Write ParaINI File.vi"("Mode"=enum16{"Read", "Write"}."Read", "Section"=w305, "Filepath"=w306, "Ctl Refnum"=w307) -> ()  [unwired: 7 in, 1 out]
                }
              }
            }
          }
          event "退出": Value Change {
            n243 = event-data() -> ()  [unwired: 1 in, 5 out]
            n244 = control-ref of="本VI"() -> (w311:refnum<vi>)
            n245 = invoke class="VI" method="FP.Close"(reference=w311) -> (reference out=w309:refnum<vi>, error out=w310:errorcluster)  [unwired: 2 in, 1 out]
            n246 = Close Reference(reference=w309, error in (no error)=w310) -> ()  [unwired: 1 out]
          }
          event "更新": Value Change {
            n247 = event-data() -> ("NewVal"=w313:bool)  [unwired: 1 in, 4 out]
            n248 = case shown="真" w313 {
              tunnel: w315 -> [_ w318]
              tunnel: w314 -> [_ w317]
              frame False {
              }
              frame True {
                n249 = for {
                  tunnel: w318 -> [w325]
                  tunnel: w317 -> [w324] mode=indexing
                  tunnel: [w323] -> w316
                  n250 = local read "产品型号"() -> (w327:string)
                  n251 = call "Read_Write ParaINI File.vi"("Mode"=enum16{"Read", "Write"}."Write", "Section"=w327, "Filepath"=w325, "Ctl Refnum"=w324) -> ("error out"=w323:errorcluster)  [unwired: 7 in]
                }
                n252 = case shown="无错误" w316 {
                  frame No Error {
                    n253 = Wait (ms)(milliseconds to wait=u32 500 ("等待时间（毫秒）")) -> ()  [unwired: 1 out]
                    n254 = One Button Dialog(message="更新成功！" ("通知内容")) -> ()  [unwired: 1 in, 1 out]
                  }
                  frame Error {
                    n255 = Wait (ms)(milliseconds to wait=u32 500 ("等待时间（毫秒）")) -> ()  [unwired: 1 out]
                    n256 = call "浮动通知.vi"("通知内容"="更新失败！") -> ()  [unwired: 11 in]
                  }
                }
              }
            }
          }
          event Panel Close {
            n257 = event-data() -> ()  [unwired: 1 in, 3 out]
          }
        }
      }
    }
  }
